vi "Create Base Icon.vi"(8 "error in (no error)":errorcluster, 10 "Label BG Color":u32(colorbox)=15925152, 11 "Label Text":string) -> (0 "error out":errorcluster, 3 "Icon.lvlclass out":refnum<class "Icon.lvclass">)   [LabVIEW 2020, in "ADAS_IO_Template_MDO.lvclass"]
uses:
  ADAS_IO_Template_MDO.lvclass
  <vilib>/LabVIEW Icon API/lv_icon/Classes/Icon/Icon.lvclass
  <vilib>/LabVIEW Icon API/API_Rectangle Dimension.ctl
  <vilib>/LabVIEW Icon API/API_Text.ctl
  <vilib>/LabVIEW Icon API/API_User Layer Data.ctl
  <vilib>/Utility/miscctls.llb/LVPoint32TypeDef.ctl
  <vilib>/picture/picture.llb/imagedata.ctl
  <vilib>/LabVIEW Icon API/LabVIEW Icon API.lvlib
panel:
  out "Picture":picture
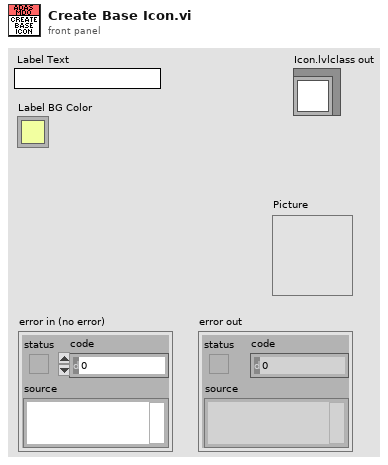
[diagram p1: front panel]
types:
  T1 = cluster{"left":i16, "top":i16, "right":i16, "bottom":i16}
  T2 = typedef "LabVIEW Icon API.lvlib/API_User Layer Data.ctl" = cluster{"Layer name":string, "Origin":T3, "Icon image data":T4}
  T3 = typedef "LVPoint32TypeDef.ctl" = cluster{"Horizontal":i32, "Vertical":i32}
  T4 = typedef "imagedata.ctl" = cluster{"image type":i32, "image depth":i32, "image":u8[], "mask":u8[], "colors":u32[], "Rectangle":cluster{"left":i16, "top":i16, "right":i16, "bottom":i16}}
  T5 = typedef "LabVIEW Icon API.lvlib/API_Text.ctl" = cluster{"Line 1 text":string, "Line 2 text":string, "Line 3 text":string, "Line 4 text":string}
  T6 = typedef "LabVIEW Icon API.lvlib/API_Rectangle Dimension.ctl" = cluster{"Width":i16, "Height":i16}
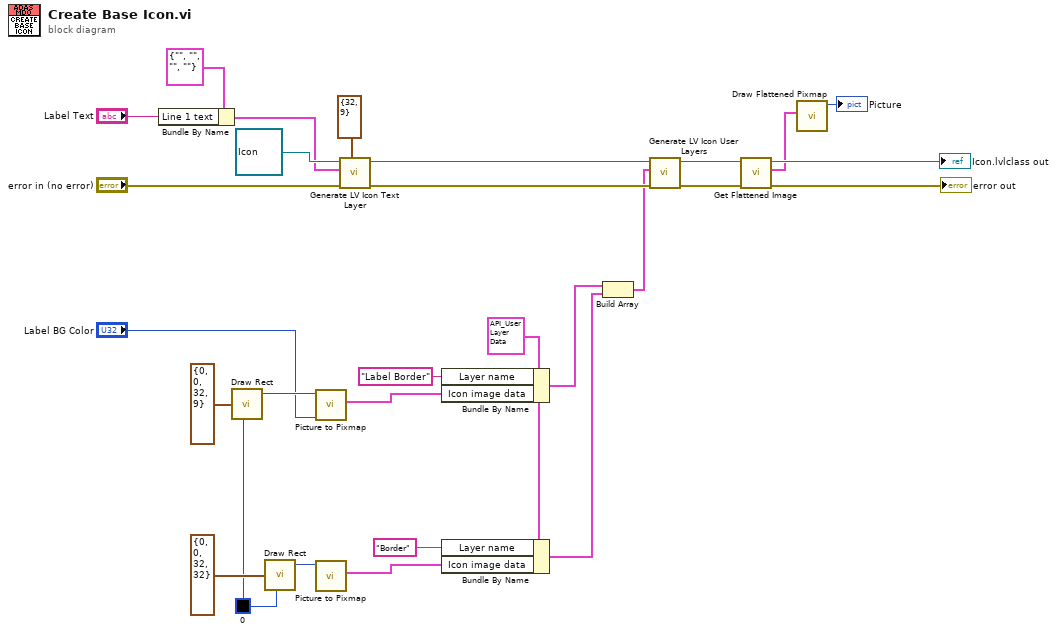
[diagram p0: block diagram]
diagram:
  w7 = u32 0 ("color(black) 2")
  w6 = T2 {"Layer name"="", "Origin"={"Horizontal"=0, "Vertical"=0}, "Icon image data"={"image type"=0, "image depth"=0, "image"=[], "mask"=[], "colors"=[], "Rectangle"={"left"=0, "top"=0, "right"=0, "bottom"=0}}} ("User layer")
  n1 = Bundle By Name(cluster=T5 {"Line 1 text"="", "Line 2 text"="", "Line 3 text"="", "Line 4 text"=""} ("Text"), "Line 1 text"="Label Text") -> (w3:T5)
  n2 = call <vilib>:"Draw Rect.vi"("rect"=T1 {"left"=0, "top"=0, "right"=32, "bottom"=9}, "color(black)"=w7) -> ("new picture"=w16:picture)  [unwired: 7 in]
  n3 = call <vilib>:"Draw Rect.vi"("rect"=T1 {"left"=0, "top"=0, "right"=32, "bottom"=32}, "color(black)"=w7) -> ("new picture"=w11:picture)  [unwired: 7 in]
  n4 = call <vilib>:"Picture to Pixmap.vi"("Background Color"="Label BG Color", "picture"=w16) -> ("image data"=w15:T4)  [unwired: 8 in, 1 out]
  n5 = call <vilib>:"Picture to Pixmap.vi"("picture"=w11) -> ("image data"=w12:T4)  [unwired: 9 in, 1 out]
  n6 = call <vilib>:"Generate LV Icon Text Layer.vi"("Rectangle dimension (32,32)"=T6 {"Width"=32, "Height"=9}, "error in (no error)"="error in (no error)", "Text"=w3, "Icon in"=refnum<class "Icon.lvclass"> refnum ("Icon.lvclass in")) -> ("error out"=w26:errorcluster, "Icon out"=w25:refnum<class "Icon.lvclass">)  [unwired: 6 in]
  n7 = Bundle By Name(cluster=w6, "Layer name"="Label Border", "Icon image data"=w15) -> (w14:T2)
  n8 = Bundle By Name(cluster=w6, "Layer name"="Border", "Icon image data"=w12) -> (w9:T2)
  n9 = Build Array(w14, w9) -> (w20:T2[])
  n10 = call <vilib>:"Generate LV Icon User Layers.vi"("error in (no error)"=w26, "User layers"=w20, "Icon in"=w25) -> ("error out"=w23:errorcluster, "Icon out"=w21:refnum<class "Icon.lvclass">)  [unwired: 7 in]
  n11 = call <vilib>:"Get Flattened Image.vi"("error in (no error)"=w23, "lv_icon.lvlib:Icon.lvclass in"=w21) -> ("error out"=→"error out":errorcluster, "Color Image"=w2:T4, "lv_icon.lvlib:Icon.lvclass out"=→"Icon.lvlclass out":refnum<class "Icon.lvclass">)  [unwired: 6 in, 1 out]
  n12 = call <vilib>:"Draw Flattened Pixmap.vi"("image data"=w2) -> ("new picture"=→"Picture":picture)  [unwired: 8 in]
